vi "Vision Lane.vi"() -> ()   [LabVIEW 2016]
uses:
  <vilib>/Platform/TimedLoop/XDataNode/timing_clust.ctl
  <vilib>/Platform/TimedLoop/XDataNode/nitl_modes.ctl
  <vilib>/Platform/TimedLoop/XDataNode/wakeup.ctl
  <vilib>/Platform/TimedLoop/XDataNode/XDataNode.xnode
  <vilib>/vision/NI_Vision_Development_Module.lvlib
  <vilib>/ptbypt/NI_PtbyPt.lvlib
  <vilib>/Platform/TimedLoop/XDataNode/XDNodeRunTimeDep.lvlib
panel:
  out "차선":dbl[][](array[numeric])
  out "Calibrated Results (Caliper 1)":sgl[][](array[numeric]) format="%.2f"
  out "Filtered image":T1(plugin-control)
  out "Original Image":T1(plugin-control)
  out "Original Image":T1(plugin-control)
  out "프레임 rate":dbl
  out "error out":errorcluster
  in  "이미지 형식":T2 items=["Grayscale (U8)", "Grayscale (I16)", "Grayscale (SGL)", "Complex (CSG)", "RGB (U32)", "HSL (U32)", "RGB (U64)", "Grayscale (U16)"]
  in  "Stop (F)":bool
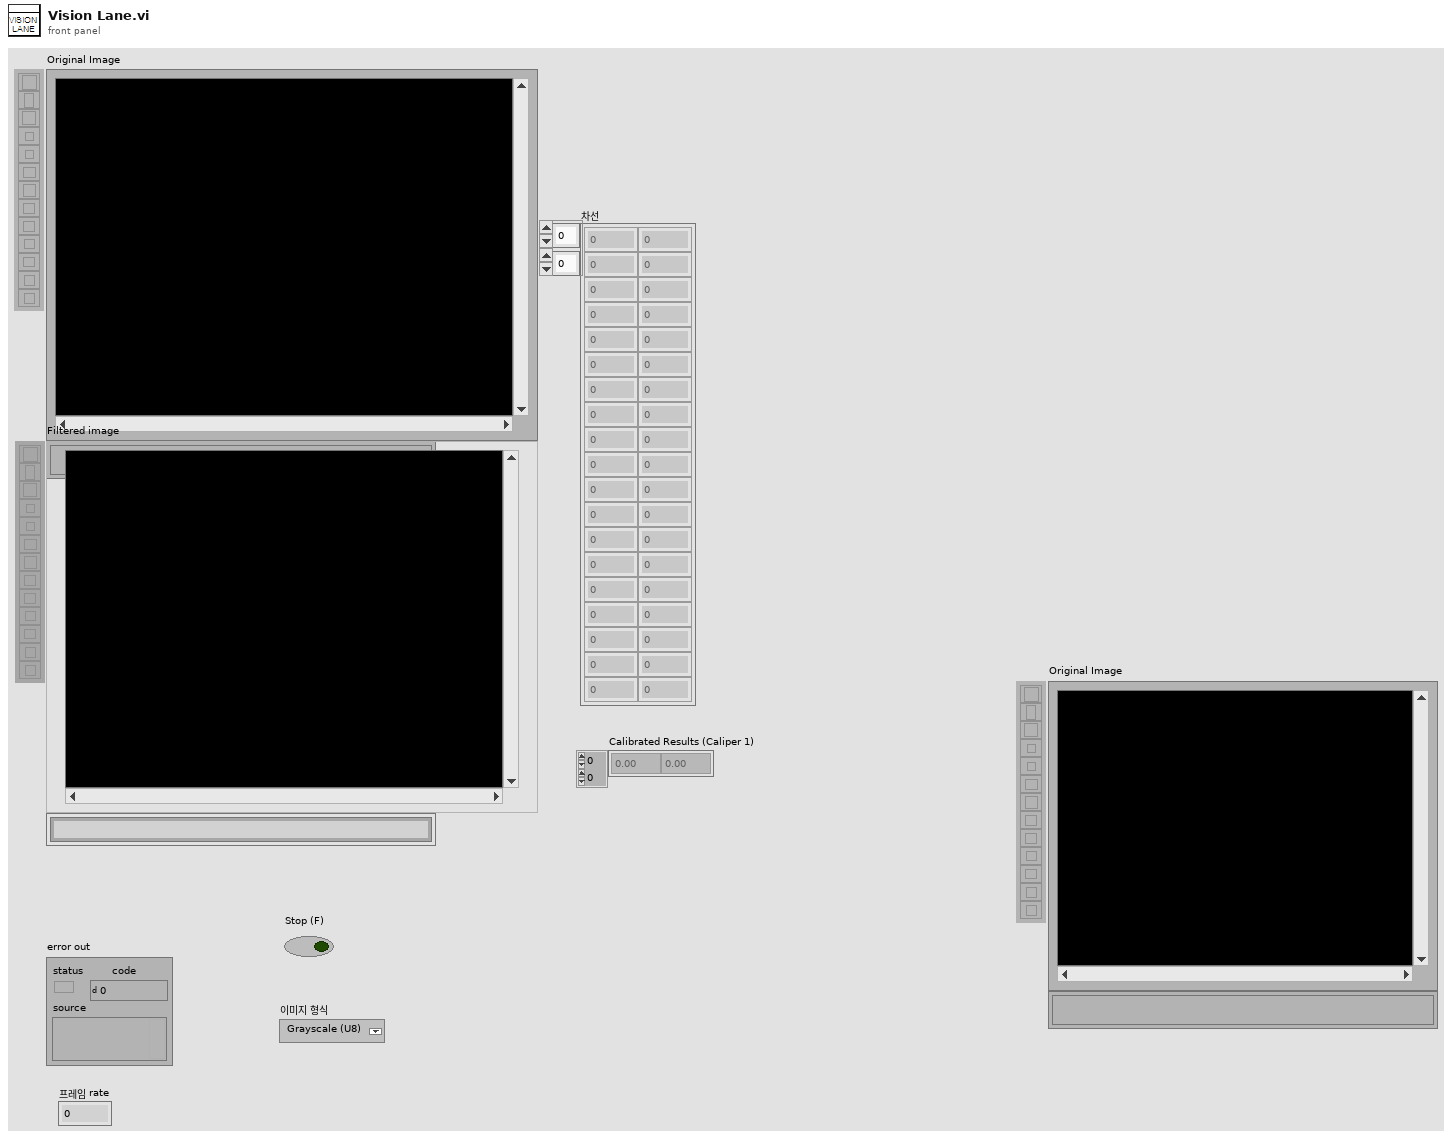
[diagram p1: front panel]
types:
  T1 = typedef "IMAQ Image.ctl" = refnum<image>
  T2 = typedef "Image Type" = u32
  T3 = typedef "XDNodeRunTimeDep.lvlib/timing_clust.ctl" = cluster{"Expected End [f-1]":u64, "Actual End [f-1]":u64, "Finished Late? [f-1]":bool, "Expected End [i-1]":u64, "Actual End [i-1]":u64, "Finished Late? [i-1]":bool, "Expected Start [i]":u64, "Actual Start [i]":u64, "Expected Start [f]":u64, "Actual Start [f]":u64, "Source Name":string, "Structure Name":string, "Period":i64, "Deadline":i64, "Offset":i64, "Start":i64, "Priority":i32, "Timeout":i32, "Mode":T4, "Wakeup Reason":T5, "Error":errorcluster, "Source Type":string, "Secondary Source Type":string, "Global End Time":u64, "Global Start Time":u64, "Frame Duration":u64, "Iteration Duration":u64, "Assigned CPU":i32, "I/O Scan Engine Mode":u32}
  T4 = typedef "XDNodeRunTimeDep.lvlib/nitl_modes.ctl" = enum32{"No Change", "Process missed periods, maintain original phase", "Discard missed periods, maintain original phase", "Process missed periods, ignore original phase", "Discard missed periods, ignore original phase"}
  T5 = typedef "XDNodeRunTimeDep.lvlib/wakeup.ctl" = enum32{"Normal", "Aborted", "Asynchronous wakeup", "Timing source error", "Timed loop error", "Timeout"}
  T6 = cluster{"Calibrated Results (Caliper 1)[0]":sgl, "Calibrated Results (Caliper 1)[1]":sgl, "Calibrated Results (Caliper 1)[2]":sgl, "Calibrated Results (Caliper 1)[3]":sgl, "Calibrated Results (Caliper 1)[4]":sgl, "Calibrated Results (Caliper 1)[5]":sgl, "Calibrated Results (Caliper 1)[6]":sgl, "Calibrated Results (Caliper 1)[7]":sgl, "Calibrated Results (Caliper 1)[8]":sgl}
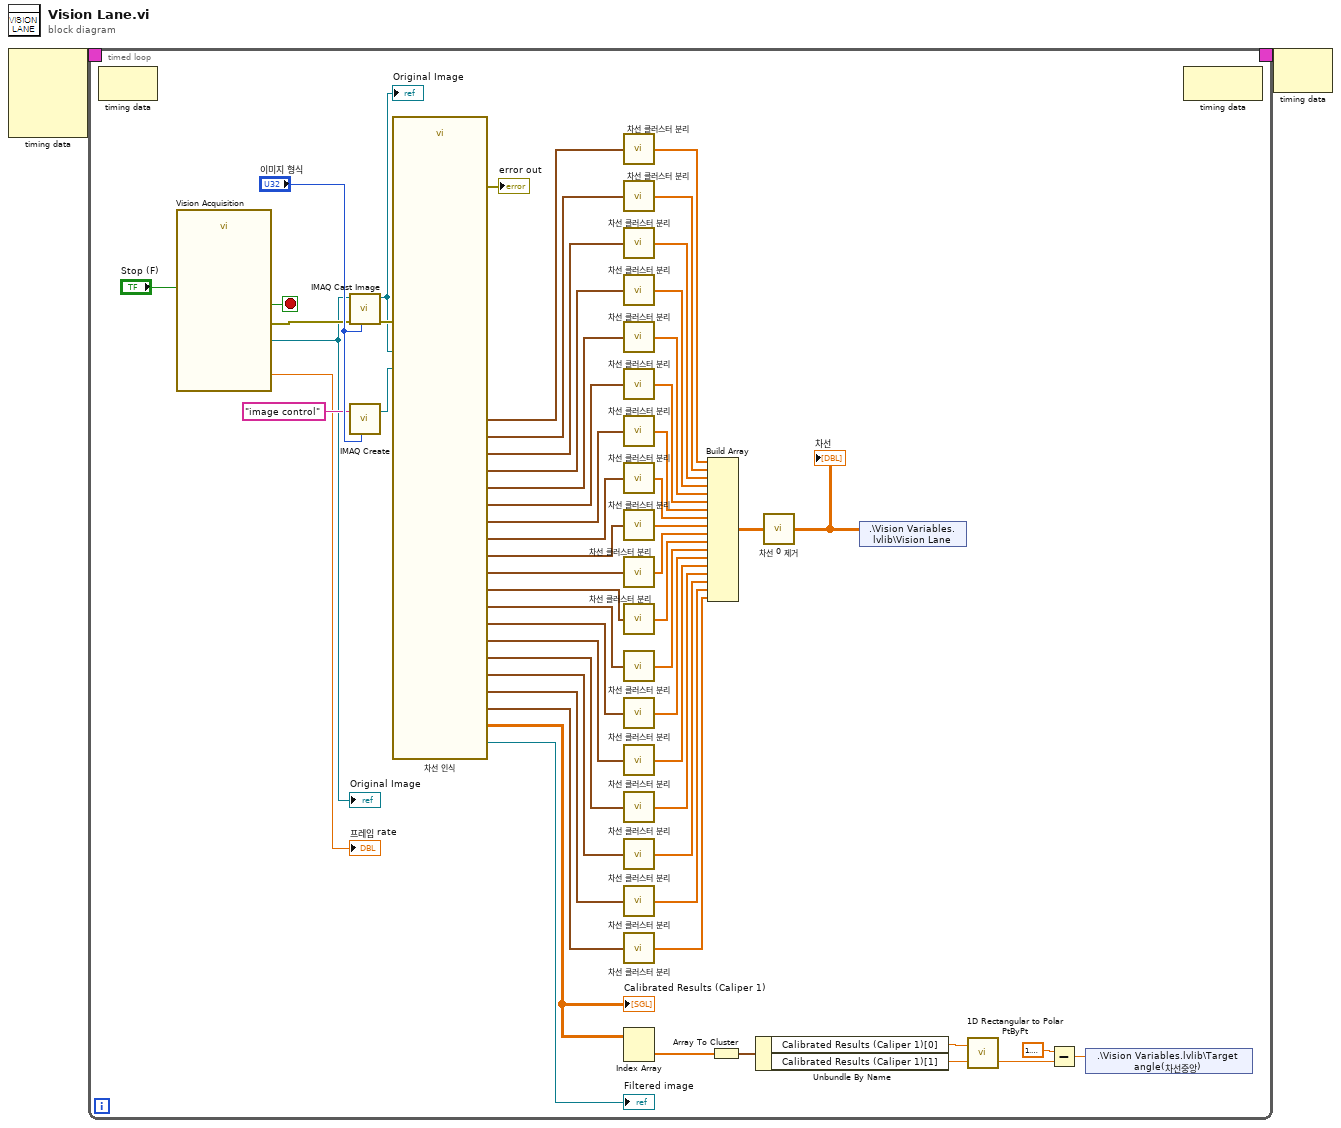
[diagram p0: block diagram]
diagram:
  n1 = node-c288() -> (w2:T3)  [unwired: 4 in]
  n2 = timed-loop {
    timing: w2 -> [_]
    timing-out: [_] -> w1
    stop <- w59 stop-if-true
    n3 = node-c288() -> ()  [unwired: 1 in, 1 out]
    n4 = call "Vision Acquisition"("Stop (F)"="Stop (F)") -> ("Image Out"=w6:T1, "Frame Rate"=→"프레임 rate":dbl, "Stopped"=w59:bool, "error out"=w56:errorcluster)  [unwired: 23 in]
    "Original Image" <- w6
    n5 = call "IMAQ Cast Image"("Image Type"="이미지 형식", "error in (no error)"=w56, "Image Src"=w6) -> ("error out"=w55:errorcluster, "Image Dst Out"=w5:T1)  [unwired: 7 in]
    "Original Image" <- w5
    n6 = call "IMAQ Create"("Image Name"="image control", "Image Type"="이미지 형식") -> ("New Image"=w4:T1)  [unwired: 3 in, 1 out]
    n7 = call "차선 인식"("Image In"=w5, "Image Dst"=w4, "error in"=w55) -> ("Calibrated Results (Caliper 1)"=w15:sgl[][], "Edges Coordinates (calibrated) (Edge Detector 21)"=w33:cluster{"X":sgl, "Y":sgl}[], "Edges Coordinates (calibrated) (Edge Detector 20)"=w34:cluster{"X":sgl, "Y":sgl}[], "Edges Coordinates (calibrated) (Edge Detector 19)"=w35:cluster{"X":sgl, "Y":sgl}[], "Edges Coordinates (calibrated) (Edge Detector 18)"=w36:cluster{"X":sgl, "Y":sgl}[], "Edges Coordinates (calibrated) (Edge Detector 17)"=w37:cluster{"X":sgl, "Y":sgl}[], "Edges Coordinates (calibrated) (Edge Detector 16)"=w38:cluster{"X":sgl, "Y":sgl}[], "Edges Coordinates (calibrated) (Edge Detector 15)"=w39:cluster{"X":sgl, "Y":sgl}[], "Edges Coordinates (calibrated) (Edge Detector 13)"=w40:cluster{"X":sgl, "Y":sgl}[], "Edges Coordinates (calibrated) (Edge Detector 12)"=w41:cluster{"X":sgl, "Y":sgl}[], "Edges Coordinates (calibrated) (Edge Detector 11)"=w42:cluster{"X":sgl, "Y":sgl}[], "Edges Coordinates (calibrated) (Edge Detector 10)"=w43:cluster{"X":sgl, "Y":sgl}[], "Edges Coordinates (calibrated) (Edge Detector 8)"=w44:cluster{"X":sgl, "Y":sgl}[], "Edges Coordinates (calibrated) (Edge Detector 7)"=w45:cluster{"X":sgl, "Y":sgl}[], "Edges Coordinates (calibrated) (Edge Detector 5)"=w46:cluster{"X":sgl, "Y":sgl}[], "Image Out"=→"Filtered image":T1, "Edges Coordinates (calibrated) (Edge Detector 1)"=w52:cluster{"X":sgl, "Y":sgl}[], "Edges Coordinates (calibrated) (Edge Detector 2)"=w50:cluster{"X":sgl, "Y":sgl}[], "Edges Coordinates (calibrated) (Edge Detector 3)"=w48:cluster{"X":sgl, "Y":sgl}[], "Edges Coordinates (calibrated) (Edge Detector 4)"=w47:cluster{"X":sgl, "Y":sgl}[], "error out"=→"error out":errorcluster)  [unwired: 2 in, 2 out]
    "Calibrated Results (Caliper 1)" <- w15
    n8 = call "차선 클러스터 분리.vi"("배열"=w52) -> ("R, Theta"=w51:dbl[])
    n9 = call "차선 클러스터 분리.vi"("배열"=w50) -> ("R, Theta"=w49:dbl[])
    n10 = call "차선 클러스터 분리.vi"("배열"=w48) -> ("R, Theta"=w32:dbl[])
    n11 = call "차선 클러스터 분리.vi"("배열"=w47) -> ("R, Theta"=w31:dbl[])
    n12 = call "차선 클러스터 분리.vi"("배열"=w46) -> ("R, Theta"=w30:dbl[])
    n13 = call "차선 클러스터 분리.vi"("배열"=w45) -> ("R, Theta"=w29:dbl[])
    n14 = call "차선 클러스터 분리.vi"("배열"=w44) -> ("R, Theta"=w28:dbl[])
    n15 = call "차선 클러스터 분리.vi"("배열"=w43) -> ("R, Theta"=w27:dbl[])
    n16 = call "차선 클러스터 분리.vi"("배열"=w42) -> ("R, Theta"=w26:dbl[])
    n17 = call "차선 클러스터 분리.vi"("배열"=w41) -> ("R, Theta"=w25:dbl[])
    n18 = call "차선 클러스터 분리.vi"("배열"=w40) -> ("R, Theta"=w24:dbl[])
    n19 = call "차선 클러스터 분리.vi"("배열"=w39) -> ("R, Theta"=w23:dbl[])
    n20 = call "차선 클러스터 분리.vi"("배열"=w38) -> ("R, Theta"=w22:dbl[])
    n21 = call "차선 클러스터 분리.vi"("배열"=w37) -> ("R, Theta"=w21:dbl[])
    n22 = call "차선 클러스터 분리.vi"("배열"=w36) -> ("R, Theta"=w19:dbl[])
    n23 = call "차선 클러스터 분리.vi"("배열"=w35) -> ("R, Theta"=w18:dbl[])
    n24 = call "차선 클러스터 분리.vi"("배열"=w34) -> ("R, Theta"=w17:dbl[])
    n25 = call "차선 클러스터 분리.vi"("배열"=w33) -> ("R, Theta"=w16:dbl[])
    n26 = Index Array(array=w15) -> (element=w14:sgl[])  [unwired: 2 in]
    n27 = Build Array(w51, w49, w32, w31, w30, w29, w28, w27, w26, w25, w24, w23, w22, w21, w19, w18, w17, w16) -> (w8:dbl[][])
    n28 = Array To Cluster(array=w14) -> (cluster=w13:T6)
    n29 = Unbundle By Name(w13) -> ("Calibrated Results (Caliper 1)[0]"=w12:sgl, "Calibrated Results (Caliper 1)[1]"=w11:sgl)
    n30 = call "차선 0 제거.vi"("추가된 배열"=w8) -> ("추가된 배열 2"=w3:dbl[][])
    "차선" <- w3
    n31 = shared-variable ".\\Vision Variables.lvlib\\Vision Lane"(w3) -> ()  [unwired: 1 in, 1 out]
    n32 = call <vilib>:"1D Rectangular to Polar PtByPt.vi"("y"=w11, "x"=w12) -> ("phase"=w9:dbl)  [unwired: 1 out]
    n33 = Subtract(x=1.5707963267948966, y=w9) -> (x-y=w7:dbl)
    n34 = shared-variable ".\\Vision Variables.lvlib\\Target angle(차선중앙)"(w7) -> ()  [unwired: 1 in, 1 out]
    n35 = node-c288() -> ()  [unwired: 1 in, 1 out]
  }
  n36 = node-c288(w1) -> ()  [unwired: 1 out]
